vi "uService GUI.vi"(8 "error in (no error)":errorcluster, 11 "uService Template in":refnum<class "DAQ Sender.lvclass">) -> (3 "uService Template out":refnum<class "DAQ Sender.lvclass">)   [LabVIEW 2020, in "TALOS.lvlib" / "DAQ Sender.lvlib" / "DAQ Sender.lvclass"]
uses:
  DAQ Sender.lvclass
  C:/LabVIEW Code/TALOS/talos/Father of all uServices/Father of all uServices/Father of all uServices.lvclass
  Ancestor/Ancestor/Ancestor.lvclass/Ancestor.ctl
  Support VIs/Substitute Error.vi
  Support VIs/Generate Error.vi
  FGV/Error Memory/Get Error Description.vi
  Support VIs/Get PC name.vi
  Ancestor/Ancestor/Read ID.vi
  Support VIs/Get Class Name.vi
  FGV/Error Memory/Error Memory Core.vi
  <vilib>/AdvancedString/Delimited String to 1D String Array.vi
  Support VIs/Circus Root Path.vi
  FGV/Error Memory/Error Crt Lvl checker.vi
  FGV/Error Memory/Error Memory Core.vi/40c8088d-b597-4017-91af-faa98e00292e.vi
  FGV/Error Memory/Error Memory Core.vi/d4a3ab98-063c-4e44-b43d-fbdcfe6c2be2.vi
  Father of all uServices/Father of all uServices/Father of all uServices.lvclass
  C:/LabVIEW Code/TALOS/builds/Actor Framework PPL/Actor Framework.lvlibp/1abvi3w/vi.lib/ActorFramework/Actor/Actor.lvclass
  builds/Actor Framework PPL/Actor Framework.lvlibp/1abvi3w/vi.lib/ActorFramework/Actor/Read Self Enqueuer.vi
  builds/Actor Framework PPL/Actor Framework.lvlibp/1abvi3w/vi.lib/ActorFramework/Stop Msg/Send Normal Stop.vi
  Support VIs/Global Memory.vi
  <vilib>/Utility/LVClass/Get LV Class Name.vi
  Support VIs/Is in Packed Library.vi
  Support VIs/TALOS Root path.vi
  Support VIs/Read CSV worksheet.vi
  Support VIs/Global Constants.vi
  <vilib>/Utility/error.llb/General Error Handler.vi
  Support VIs/Error Log.vi
  Ancestor/Ancestor/Ancestor.lvclass
  <vilib>/Comparison/Equal/Equal Functor/Equal Functor.lvclass
panel:
  out "Safe Mode":bool
  in  "Stop":bool
  out "uService ID":string
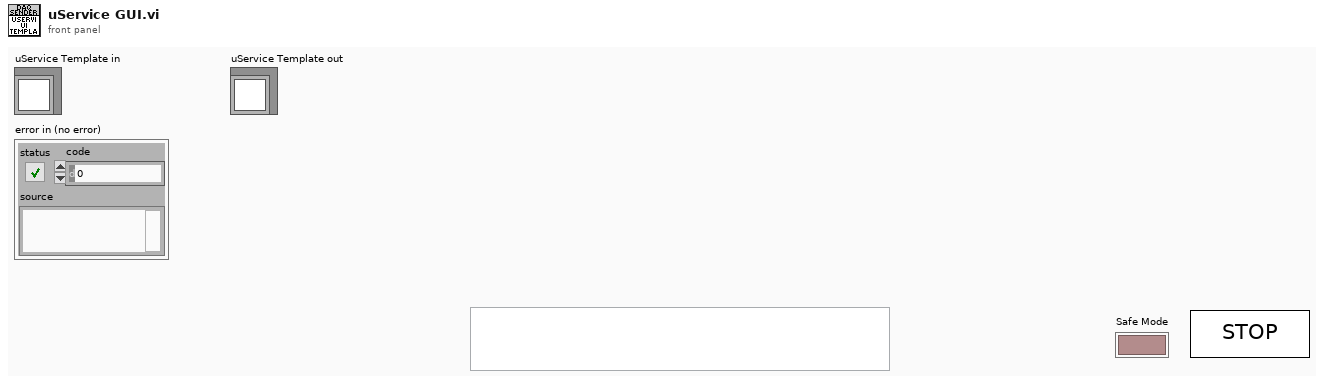
[diagram p1: front panel]
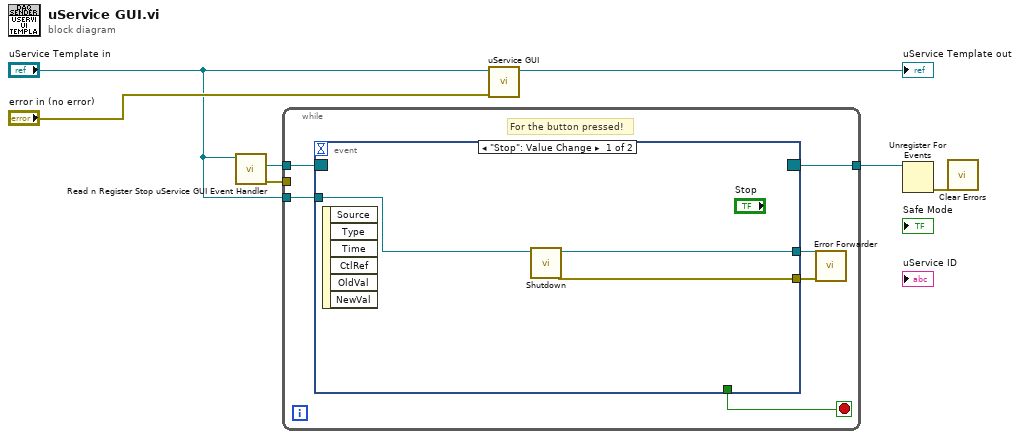
[diagram p0: block diagram]
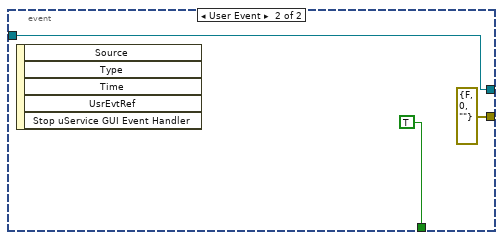
[diagram p2: hidden frame]
diagram:
  n1 = call-dynamic "Read n Register Stop uService GUI Event Handler .vi"("uService Template in"="uService Template in") -> ("error out"=w4:errorcluster, "Stop uService GUI Event Ref"=w3:refnum<event-registration>)  [unwired: 8 in, 1 out]
  n2 = while {
    tunnel: [w13] -> w5
    tunnel: w4 -> [_]
    tunnel: "uService Template in" -> [w11]
    tunnel: w3 -> [w10]
    stop <- w12 stop-if-true
    # "For the button pressed!"
    n3 = event shown="[0] \"Stop\": Value Change" {
      selector: w10 -> [_ _]
      dyn-events: [_ _] -> w13
      timeout: _ -> [_ _]
      tunnel: w11 -> [w16 w18]
      tunnel: [_ TRUE] -> w12
      tunnel: [w15 w18] -> w9
      tunnel: [w14 errorcluster {"status"=FALSE, "code"=0, "source"=""} ("error out")] -> w8
      event "Stop": Value Change {
        n4 = event-data() -> ()  [unwired: 1 in, 6 out]
        n5 = call "Shutdown.vi"("Father of all uServices in"=w16) -> ("error out"=w14:errorcluster, "Father of all uServices out"=w15:refnum<class "DAQ Sender.lvclass">)  [unwired: 9 in]
      }
      event User Event {
        n6 = event-data() -> ()  [unwired: 1 in, 5 out]
      }
    }
    n7 = call "Error Forwarder.vi"("error in (no error)"=w8, "Father of all uServices in"=w9) -> ()  [unwired: 10 in]
  }
  n8 = call-parent "uService GUI.vi"("error in (no error)"="error in (no error)", "uService Template in"="uService Template in") -> ("uService Template out"=→"uService Template out":refnum<class "DAQ Sender.lvclass">)  [unwired: 9 in]
  n9 = Unregister For Events(event registration refnum=w5) -> (error out=w1:errorcluster)  [unwired: 1 in]
  n10 = call <vilib>:"Clear Errors.vi"("error in (no error)"=w1) -> ()  [unwired: 5 in, 2 out]
